vi "Main.vi"(11 "Module Admin":refnum<class "Delacor_lib_QMH_Module Admin.lvclass">) -> ()   [LabVIEW 2020, in "Control Property Tree.lvlib"]
doc: "This template is based off of the Queued Message Handler design pattern and the Queued Message Handler project template that ships with LabVIEW.\n\nThe main difference is that the queue is private to this module and communication between modules is performed via Broadcast and Request events.\n\nRequest events are wrapped in public API methods and are handled in the Event Handling Loop (EHL) of this VI. Any module can register for Broadcast events sent by this module. The EHL generates messages based on user interface actions.\n\nThe Message Handling Loop (MHL) processes messages generated by the EHL, or by other messages. The messages are string values, so new messages can be added easily to the Message Cases case structure in the MHL. Each message cluster can also provide an optional value for Message Data, which is a variant that can be converted to whatever message-specific data is required.\n_____\nBased on Delacor QMH Project Template 5.0.0.82."
uses:
  Control Property Tree.lvlib
  <vilib>/Delacor/Delacor QMH/Libraries/Module Admin_class/Delacor_lib_QMH_Module Admin.lvclass
  Module Data--cluster.ctl
  <vilib>/Delacor/Delacor QMH/Libraries/Message Queue_class/Delacor_lib_QMH_Message Queue.lvclass/Delacor_lib_QMH_Message Queue.ctl
  Stop Argument--cluster.ctl
  <vilib>/Delacor/Delacor QMH/Libraries/Module Admin_class/Delacor_lib_QMH_Module Admin.lvclass/Delacor_lib_QMH_Module Admin.ctl
  Load Available PN Argument--cluster.ctl
  <vilib>/Utility/miscctls.llb/LVPointTypeDef.ctl
  <vilib>/Delacor/Delacor QMH/Libraries/Message Queue_class/Delacor_lib_QMH_Enqueue Message (Single).vi
  <vilib>/Delacor/Delacor QMH/Libraries/Module Admin_class/Delacor_lib_QMH_Get External Launch.vi
  <vilib>/Utility/error.llb/Error Cluster From Error Code.vi
  <vilib>/ErrorRing/Error Ring.xnode
  <vilib>/Delacor/Delacor QMH/Libraries/Message Queue_class/Delacor_lib_QMH_Message Queue.lvclass
panel:
  in  "Add Control":bool
  in  "Remove Control":bool
  in  "List of Controls":string[](tree)
  in  "List of Properties":string(tree)
  in  "Simulate MHL Error":bool
  in  "Simulate EHL Error":bool
  out "error out":errorcluster
  out "Status":string
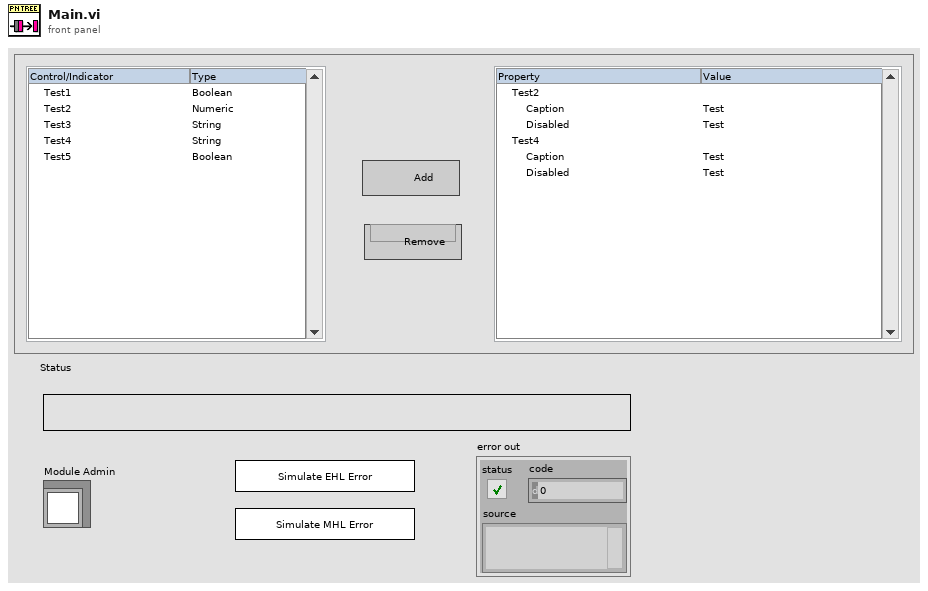
[diagram p1: front panel]
types:
  T1 = typedef "Control Property Tree.lvlib/Request Events--cluster.ctl" = cluster{"Stop Module":refnum<user-event>, "Show Panel":refnum<user-event>, "Hide Panel":refnum<user-event>, "Get Module Execution Status":refnum<user-event>, "Show Diagram":refnum<user-event>, "Load List of Controls":refnum<user-event>, "Load Available PN":refnum<user-event>}
  T2 = typedef "Control Property Tree.lvlib/Module Data--cluster.ctl" = cluster{"Status":string, "UI Ctrls":cluster{"Ctrl Names":string[], "Ctrl Types":string[], "Ctrl Tags":string[]}, "Selected Ctrls":cluster{"Ctrl Names":string[], "Ctrl Types":string[], "Ctrl Tags":string[]}, "Ctrl Properties":map{string, cluster{"Name":string, "Type":string, "Properties":cluster{"Property name":string, "Property value":variant}[]}}, "Ctrl Properties Template":map{string, cluster{"Property name":string, "Property value":variant}[]}}
  T3 = enum32{"invalid lock state", "Not Locked", "Locked (No Password)", "Password-protected"}
  T4 = typedef "Control Property Tree.lvlib/Stop Argument--cluster.ctl" = cluster{"Origin":string, "Exit via Stop Module Req?":bool, "Wait for Module to stop?":bool}
  T5 = typedef "Control Property Tree.lvlib/Load Available PN Argument--cluster.ctl" = cluster{"Boolean":bool}
  T6 = typedef "LVPointTypeDef.ctl" = cluster{"Horizontal":i16, "Vertical":i16}
  T7 = enum32{"Invalid", "Standard", "Closed", "Hidden", "Minimized", "Maximized"}
  T8 = cluster{"Ctrl Names":string[], "Ctrl Types":string[], "Ctrl Tags":string[]}
  T9 = cluster{"Property name":string, "Property value":variant}[]
  T10 = map{string, cluster{"Property name":string, "Property value":variant}[]}
  T11 = cluster{"Left Cell String":string, "Child Text":string[], "Child Tag":string, "Item Indent":i32, "Child Only?":bool, "Glyph Index":i32}[]
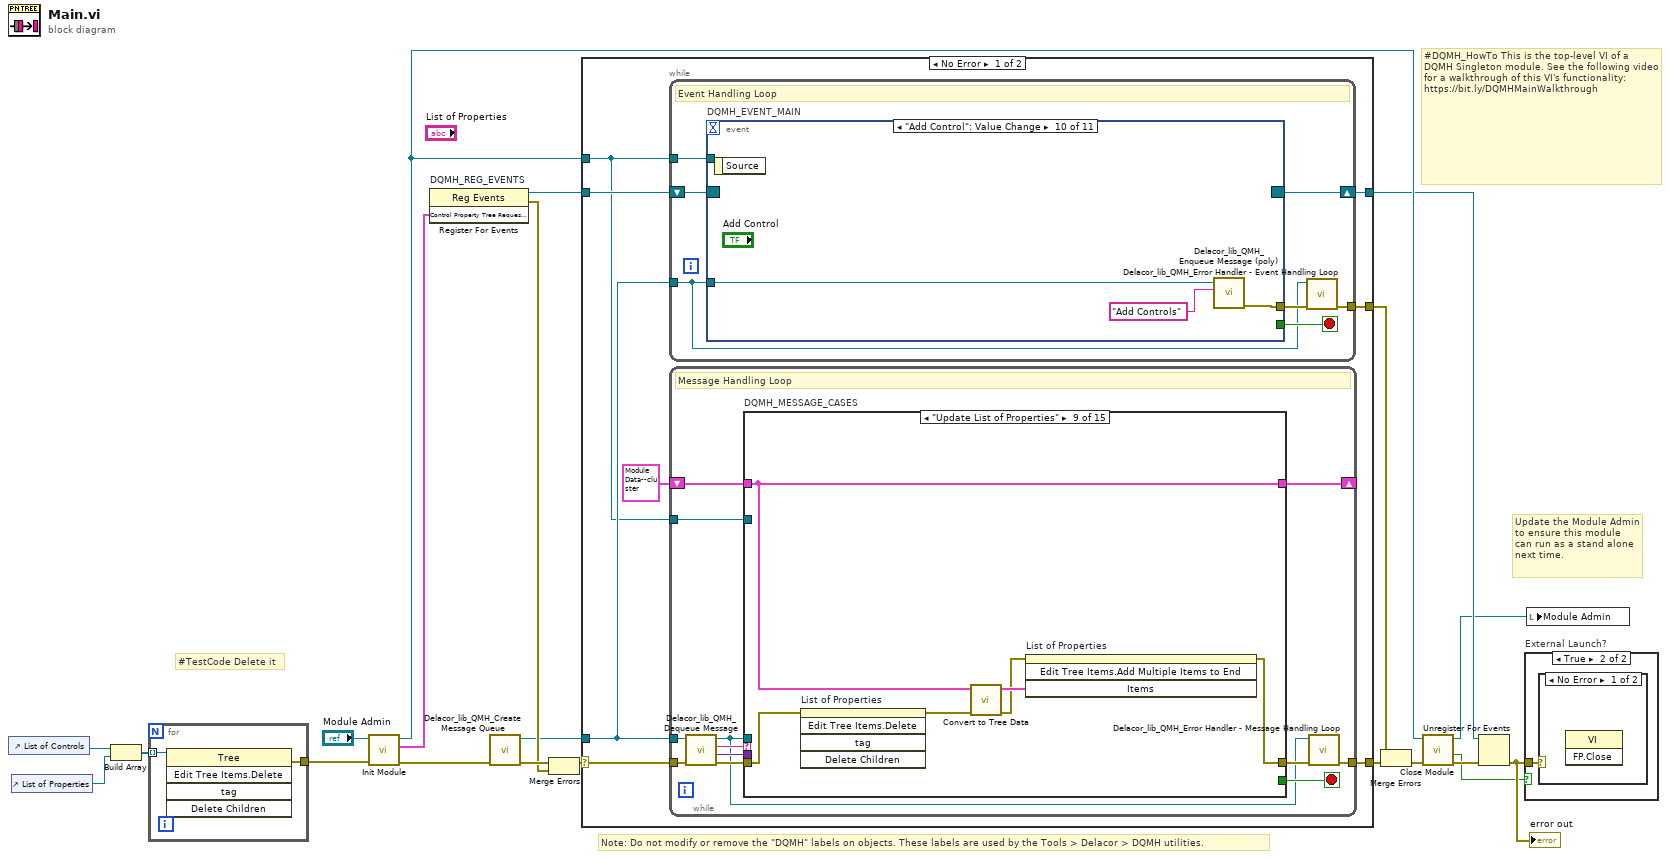
[diagram p0: block diagram]
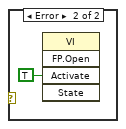
[diagram p3: hidden frame]
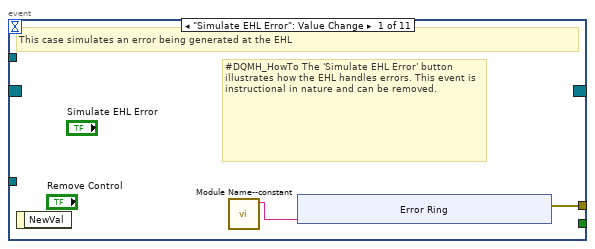
[diagram p4: hidden frame]
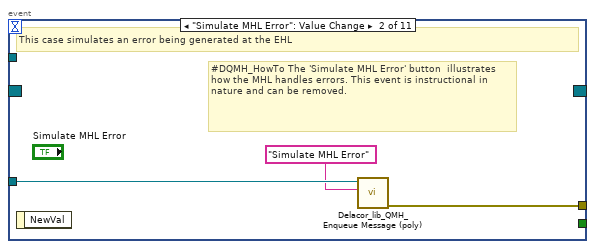
[diagram p5: hidden frame]
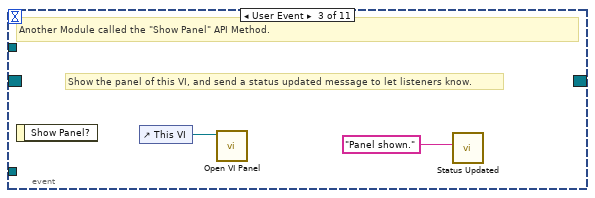
[diagram p6: hidden frame]
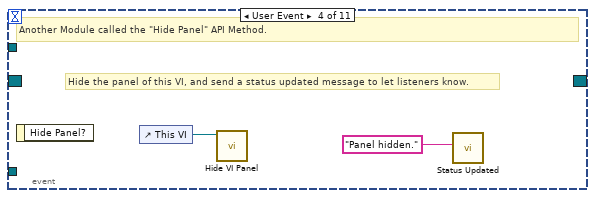
[diagram p7: hidden frame]
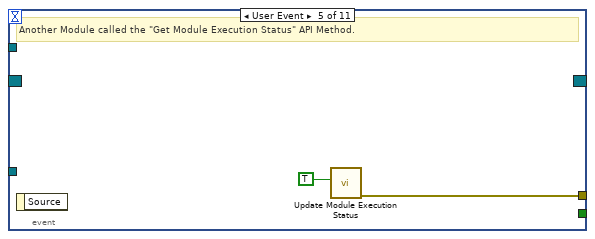
[diagram p8: hidden frame]
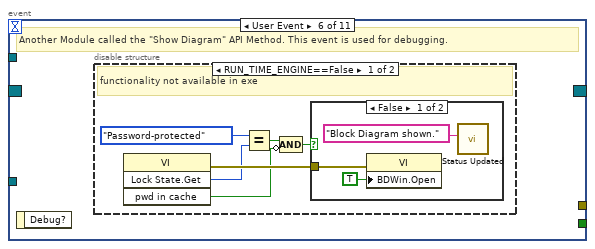
[diagram p9: hidden frame]
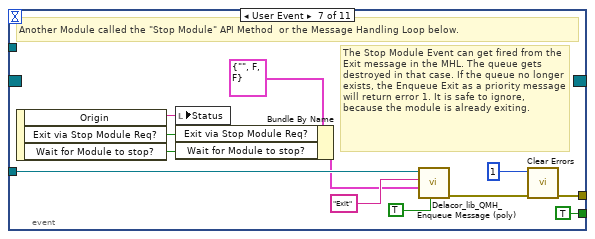
[diagram p12: hidden frame]
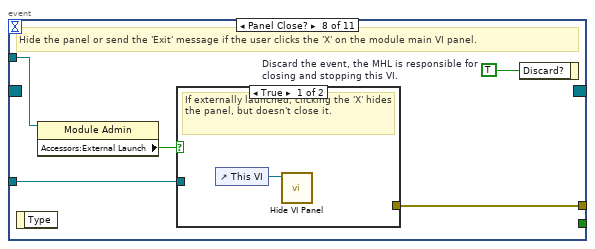
[diagram p13: hidden frame]
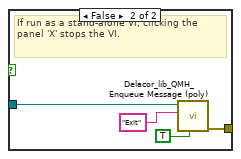
[diagram p14: hidden frame]
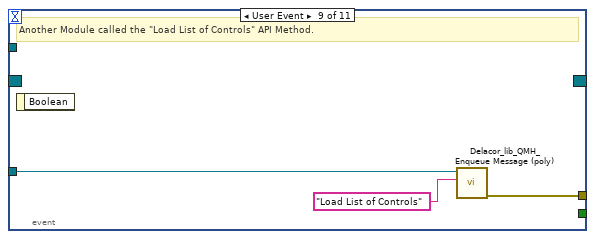
[diagram p15: hidden frame]
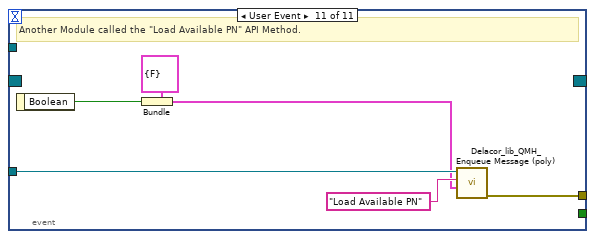
[diagram p16: hidden frame]
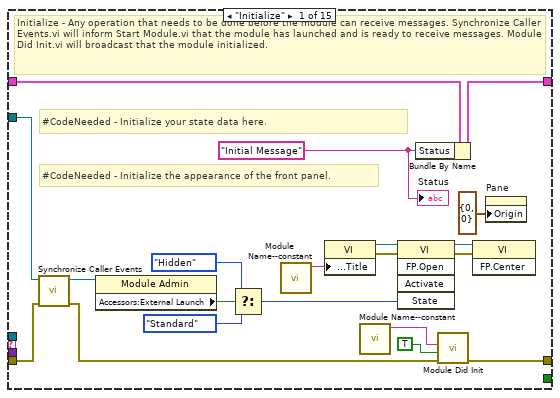
[diagram p17: hidden frame]
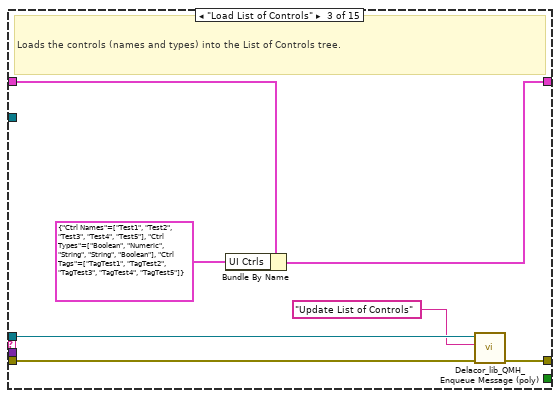
[diagram p19: hidden frame]
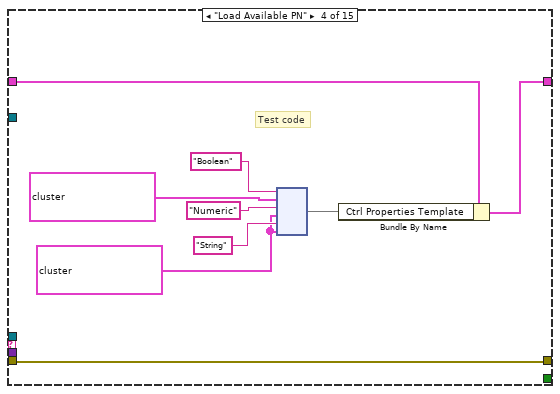
[diagram p20: hidden frame]
diagram:
  # "#TestCode Delete it"
  # "#DQMH_HowTo This is the top-level VI of a DQMH Singleton module. See the following video for a walkthrough of this VI's functionality: https://bit.ly/DQMHMainWalkthrough"
  # "Note: Do not modify or remove the \"DQMH\" labels on objects. These labels are used by the Tools > Delacor > DQMH utilities."
  # "Update the Module Admin to ensure this module can run as a stand alone next time."
  n1 = control-ref of="List of Controls"() -> (w3:refnum<vi>)
  n2 = control-ref of="List of Properties"() -> (w2:refnum<vi>)
  n3 = Build Array(w3, w2) -> (w1:refnum<vi>[])
  n4 = for {
    tunnel: [w23] -> w4
    tunnel: w1 -> [w22] mode=indexing
    n5 = invoke on="Invoke Node" class="Tree" method="Edit Tree Items.Delete"(reference=w22) -> (error out=w23:errorcluster)  [unwired: 4 in, 4 out]
  }
  n6 = call "Init Module.vi"("error in (no error)"=w4, "Singleton Module Admin in"="Module Admin") -> ("error out"=w20:errorcluster, "Control Property Tree Request Events"=w9:T1, "Singleton Module Admin out"=w12:refnum<class "Delacor_lib_QMH_Module Admin.lvclass">)  [unwired: 7 in]
  n7 = register-events "DQMH_REG_EVENTS"(w9) -> (reference out=w10:refnum<event-registration>, error out=w13:errorcluster)  [unwired: 2 in]
  n8 = call <vilib>:"Delacor_lib_QMH_Create Message Queue.vi"("error in (no error)"=w20) -> ("error out"=w15:errorcluster, "Message Queue"=w8:refnum<class "Delacor_lib_QMH_Message Queue.lvclass">)  [unwired: 9 in]
  n9 = Merge Errors(w15, w13) -> (w14:errorcluster)
  n10 = case shown="No Error" w14 {
    selector: w14 -> [w29 w246]
    tunnel: [w31 w245] -> w21
    tunnel: [w28 w251] -> w11
    tunnel: w10 -> [w26 w251]
    tunnel: w8 -> [w25 w244]
    tunnel: [w30 _] -> w18
    tunnel: w12 -> [w24 w247]
    frame No Error {
      n11 = while {
        tunnel: w25 -> [w32]
        shift-right: [w35] -> w28
        shift-left: w26 -> [w36]
        tunnel: [w37] -> w30
        tunnel: w24 -> [w33]
        stop <- w34 stop-if-true
        # "Event Handling Loop"
        n12 = event "DQMH_EVENT_MAIN" shown="[9] \"Add Control\": Value Change" {
          selector: w36 -> [_ _ _ _ _ _ _ _ _ _ _]
          dyn-events: [_ _ _ _ _ _ _ _ _ _ _] -> w35
          timeout: _ -> [_ _ _ _ _ _ _ _ _ _ _]
          tunnel: [_ _ _ _ _ _ TRUE ("Discard?") _ _ _ _] -> w34
          tunnel: w32 -> [_ w49 _ _ _ _ w73 w80 w90 w92 w99]
          tunnel: [w40 w50 _ _ w56 _ w76 w82 w88 w91 w94] -> w38
          tunnel: w33 -> [_ _ _ _ _ _ _ w79 _ _ _]
          event "Simulate EHL Error": Value Change {
            # "#DQMH_HowTo The 'Simulate EHL Error' button  illustrates how the EHL handles errors. This event is instructional in nature and can be removed."
            # "This case simulates an error being generated at the EHL"
            n13 = event-data() -> ()  [unwired: 1 in, 1 out]
            n14 = call "Module Name--constant.vi"() -> ("Module Name"=w39:string)  [unwired: 11 in]
            n15 = xnode "Error Ring"("parameter 0"=w39) -> ("error out"=w40:errorcluster)
          }
          event "Simulate MHL Error": Value Change {
            # "#DQMH_HowTo The 'Simulate MHL Error' button  illustrates how the MHL handles errors. This event is instructional in nature and can be removed."
            # "This case simulates an error being generated at the EHL"
            n16 = event-data() -> ()  [unwired: 1 in, 1 out]
            n17 = call-poly <vilib>:"Delacor_lib_QMH_Enqueue Message (poly).vi"("Message"="Simulate MHL Error", "Message Queue in"=w49) -> ("error out"=w50:errorcluster)  [unwired: 8 in, 1 out]
          }
          event User Event {
            # "Show the panel of this VI, and send a status updated message to let listeners know."
            # "Another Module called the \"Show Panel\" API Method."
            n18 = event-data() -> ()  [unwired: 1 in, 1 out]
            n19 = control-ref of="This VI"() -> (w52:refnum<vi>)
            n20 = call "Open VI Panel.vi"("VI"=w52) -> ()  [unwired: 10 in, 1 out]
            n21 = call "Status Updated.vi"("Status"="Panel shown." ("format string")) -> ()  [unwired: 10 in, 1 out]
          }
          event User Event {
            # "Hide the panel of this VI, and send a status updated message to let listeners know."
            # "Another Module called the \"Hide Panel\" API Method."
            n22 = event-data() -> ()  [unwired: 1 in, 1 out]
            n23 = control-ref of="This VI"() -> (w54:refnum<vi>)
            n24 = call "Hide VI Panel.vi"("VI"=w54) -> ()  [unwired: 10 in, 1 out]
            n25 = call "Status Updated.vi"("Status"="Panel hidden." ("format string")) -> ()  [unwired: 10 in, 1 out]
          }
          event User Event {
            # "Another Module called the \"Get Module Execution Status\" API Method."
            n26 = event-data() -> ()  [unwired: 1 in, 1 out]
            n27 = call "Update Module Execution Status.vi"("Running?"=TRUE) -> ("error out"=w56:errorcluster)  [unwired: 10 in]
          }
          event User Event {
            # "Another Module called the \"Show Diagram\" API Method. This event is used for debugging."
            n28 = event-data() -> ()  [unwired: 1 in, 1 out]
            n29 = disable-structure shown="RUN_TIME_ENGINE==False" {
              frame condition #0 (active) {
                # "functionality not available in exe"
                n30 = invoke class="VI" method="Lock State.Get"() -> (error out=w62:errorcluster, "Get Lock State"=w61:T3, "pwd in cache"=w58:bool)  [unwired: 4 in, 1 out]
                n31 = Equal?(x=T3."Password-protected", y=w61) -> (x = y?=w59:bool)
                n32 = Compound Arithmetic op=AND(w59, invert w58) -> (w57:bool)
                n33 = case shown="False" w57 {
                  tunnel: w62 -> [w65 _]
                  frame False {
                    n34 = property class="VI"(error in=w65, "BDWin.Open"=TRUE ("Block Diagram Window:Open")) -> ()  [unwired: 1 in, 2 out]
                    n35 = call "Status Updated.vi"("Status"="Block Diagram shown." ("format string")) -> ()  [unwired: 10 in, 1 out]
                  }
                  frame True {
                    # "Password-protected VI, and the password is not in the cache. Do not show the diagram."
                  }
                }
              }
              frame condition #1 {
              }
            }
          }
          event User Event {
            # "The Stop Module Event can get fired from the Exit message in the MHL. The queue gets destroyed in that case. If the queue no longer exists, the Enqueue Exit as a priority message will return error 1. It is safe to ignore, because the module is already exiting."
            # "Another Module called the \"Stop Module\" API Method  or the Message Handling Loop below."
            n36 = event-data() -> ("Origin"=w72:string, "Exit via Stop Module Req?"=w68:bool, "Wait for Module to stop?"=w67:bool)  [unwired: 1 in]
            n37 = local write "Status"(w72) -> ()
            n38 = Bundle By Name(cluster=T4 {"Origin"="", "Exit via Stop Module Req?"=FALSE, "Wait for Module to stop?"=FALSE} ("Stop Argument"), "Exit via Stop Module Req?"=w68, "Wait for Module to stop?"=w67) -> (w66:T4)
            n39 = call-poly <vilib>:"Delacor_lib_QMH_Enqueue Message (poly).vi"("Priority Message? (F)"=TRUE, "Message Data"=w66, "Message"="Exit", "Message Queue in"=w73) -> ("error out"=w77:errorcluster)  [unwired: 6 in, 1 out]
            n40 = call <vilib>:"Clear Errors.vi"("error in (no error)"=w77, "specific error code to clear (0: all)"=1) -> ("error out"=w76:errorcluster)  [unwired: 4 in, 1 out]
          }
          event Panel Close? {
            w81 = TRUE  # Discard the event, the MHL is responsible for closing and stopping this VI.
            # "Hide the panel or send the 'Exit' message if the user clicks the 'X' on the module main VI panel."
            n41 = event-data() -> ()  [unwired: 1 in, 1 out]
            n42 = property class="Module Admin"(reference=w79) -> ("Accessors:External Launch"=w78:bool)  [unwired: 1 in, 2 out]
            n43 = case shown="True" w78 {
              tunnel: w80 -> [_ w86]
              tunnel: [_ w87] -> w82
              frame True {
                # "If externally launched, clicking the 'X' hides the panel, but doesn't close it."
                n44 = control-ref of="This VI"() -> (w83:refnum<vi>)
                n45 = call "Hide VI Panel.vi"("VI"=w83) -> ()  [unwired: 10 in, 1 out]
              }
              frame False {
                # "If run as a stand-alone VI, clicking the panel 'X' stops the VI."
                n46 = call-poly <vilib>:"Delacor_lib_QMH_Enqueue Message (poly).vi"("Priority Message? (F)"=TRUE, "Message"="Exit", "Message Queue in"=w86) -> ("error out"=w87:errorcluster)  [unwired: 7 in, 1 out]
              }
            }
            n47 = event-data("Discard?"=w81) -> ()  [unwired: 1 in, 1 out]
          }
          event User Event {
            # "Another Module called the \"Load List of Controls\" API Method."
            n48 = event-data() -> ()  [unwired: 1 in, 1 out]
            n49 = call-poly <vilib>:"Delacor_lib_QMH_Enqueue Message (poly).vi"("Message"="Load List of Controls", "Message Queue in"=w90) -> ("error out"=w88:errorcluster)  [unwired: 8 in, 1 out]
          }
          event "Add Control": Value Change {
            n50 = event-data() -> ()  [unwired: 1 in, 1 out]
            n51 = call-poly <vilib>:"Delacor_lib_QMH_Enqueue Message (poly).vi"("Message"="Add Controls", "Message Queue in"=w92) -> ("error out"=w91:errorcluster)  [unwired: 8 in, 1 out]
          }
          event User Event {
            # "Another Module called the \"Load Available PN\" API Method."
            n52 = event-data() -> ("Boolean"=w95:bool)  [unwired: 1 in]
            n53 = Bundle(cluster=T5 {"Boolean"=FALSE} ("Load Available PN Argument"), "Boolean"=w95) -> (w96:T5)
            n54 = call-poly <vilib>:"Delacor_lib_QMH_Enqueue Message (poly).vi"("Message Data"=w96, "Message"="Load Available PN", "Message Queue in"=w99) -> ("error out"=w94:errorcluster)  [unwired: 7 in, 1 out]
          }
        }
        n55 = call-dynamic "Delacor_lib_QMH_Error Handler - Event Handling Loop.vi"("error in (no error)"=w38, "Message Queue in"=w32) -> ("dup error in"=w37:errorcluster)  [unwired: 8 in, 1 out]
      }
      n56 = while {
        tunnel: w25 -> [w102]
        shift-right: [w106] -> _
        shift-left: T2 {"Status"="", "UI Ctrls"={"Ctrl Names"=[], "Ctrl Types"=[], "Ctrl Tags"=[]}, "Selected Ctrls"={"Ctrl Names"=[], "Ctrl Types"=[], "Ctrl Tags"=[]}, "Ctrl Properties"={}, "Ctrl Properties Template"={}} ("Data Cluster") -> [w107]
        tunnel: w29 -> [w110]
        tunnel: [w108] -> w31
        tunnel: w24 -> [w100]
        stop <- w105 stop-if-true
        # "Message Handling Loop"
        n57 = call-dynamic "Delacor_lib_QMH_Dequeue Message.vi"("error in (no error)"=w110, "Message Queue in"=w102) -> ("error out"=w109:errorcluster, "Message Data"=w103:variant, "Message"=w104:string, "Message Queue out"=w101:refnum<class "Delacor_lib_QMH_Message Queue.lvclass">)  [unwired: 6 in]
        n58 = case "DQMH_MESSAGE_CASES" shown="\"Update List of Properties\"" w104 {
          selector: w104 -> [_ _ _ _ _ _ _ _ _ _ _ _ _ _ w231]
          tunnel: w101 -> [_ _ w135 _ _ w155 _ w171 _ _ _ _ w201 w223 _]
          tunnel: w109 -> [w129 w133 w137 w141 w151 w160 w164 w170 w176 w183 w185 w190 w208 w229 w233]
          tunnel: [w127 w133 w136 w141 w154 w156 w163 w169 w180 w182 w185 w189 w204 w226 w234] -> w111
          tunnel: w107 -> [w118 w132 w140 w143 w153 w162 w167 w174 w179 w181 w184 w187 w203 w222 w232]
          tunnel: [w117 w132 w138 w142 w153 w162 w166 w173 w179 w181 w184 w187 w203 w222 w232] -> w106
          tunnel: [_ _ _ _ _ _ _ _ _ _ _ _ _ w221 _] -> w105
          tunnel: w103 -> [_ _ _ _ _ _ _ _ _ _ _ _ w202 w220 _]
          tunnel: w100 -> [w119 _ _ _ _ _ _ _ _ _ _ _ w200 w215 _]
          frame "Initialize" {
            w112 = "Initial Message" ("Initial Message")
            # "#CodeNeeded - Initialize the appearance of the front panel."
            # "#CodeNeeded - Initialize your state data here."
            # "Initialize - Any operation that needs to be done before the module can receive messages. Synchronize Caller Events.vi will inform Start Module.vi that the module has launched and is ready to receive messages. Module Did Init.vi will broadcast that the module initialized."
            n59 = call "Synchronize Caller Events.vi"("error in (no error)"=w129, "Singleton Module Admin in"=w119) -> ("error out"=w128:errorcluster, "Singleton Module Admin out"=w114:refnum<class "Delacor_lib_QMH_Module Admin.lvclass">)  [unwired: 8 in]
            n60 = property class="Module Admin"(reference=w114) -> ("Accessors:External Launch"=w123:bool)  [unwired: 1 in, 2 out]
            n61 = Select(t=T7."Hidden" ("State"), s=w123, f=T7."Standard" ("State")) -> (s? t:f=w120:T7)
            n62 = call "Module Name--constant.vi"() -> ("Module Name"=w126:string)  [unwired: 11 in]
            n63 = property class="VI"("Front Panel.Title"=w126) -> (reference out=w125:refnum<vi>, error out=w131:errorcluster)  [unwired: 2 in]
            n64 = call "Module Name--constant.vi"() -> ("Module Name"=w115:string)  [unwired: 11 in]
            n65 = invoke class="VI" method="FP.Open"(reference=w125, error in=w131, "State"=w120) -> (reference out=w124:refnum<vi>, error out=w130:errorcluster)  [unwired: 2 in, 3 out]
            n66 = Bundle By Name(cluster=w118, "Status"=w112) -> (w117:T2)
            n67 = call "Module Did Init.vi"("error in (no error)"=w128, "Initialized?"=TRUE, "Origin"=w115) -> ("error out"=w127:errorcluster)  [unwired: 8 in]
            n68 = invoke class="VI" method="FP.Center"(reference=w124, error in=w130) -> ()  [unwired: 1 in, 3 out]
            n69 = property on="Pane" class="Pane"("Origin"=T6 {"Horizontal"=0, "Vertical"=0}) -> ()  [unwired: 2 in, 2 out]
            "Status" <- w112
          }
          frame "--- Module Specific ---" {
            # "Separator -- The following cases handle messages specific to this Module."
          }
          frame "Load List of Controls" {
            # "Loads the controls (names and types) into the List of Controls tree."
            n70 = Bundle By Name(cluster=w140, "UI Ctrls"=T8 {"Ctrl Names"=["Test1", "Test2", "Test3", "Test4", "Test5"], "Ctrl Types"=["Boolean", "Numeric", "String", "String", "Boolean"], "Ctrl Tags"=["TagTest1", "TagTest2", "TagTest3", "TagTest4", "TagTest5"]}) -> (w138:T2)
            n71 = call-poly <vilib>:"Delacor_lib_QMH_Enqueue Message (poly).vi"("error in (no error)"=w137, "Message"="Update List of Controls", "Message Queue in"=w135) -> ("error out"=w136:errorcluster)  [unwired: 7 in, 1 out]
          }
          frame "Load Available PN" {
            w145 = T9 [{"Property name"="Caption", "Property value"=variant}, {"Property name"="Disabled", "Property value"=variant}] ("Properties")
            # "Test code"
            n72 = node("Boolean" ("key"), T9 [{"Property name"="Caption", "Property value"=variant}, {"Property name"="Disabled", "Property value"=variant}, {"Property name"="Blinking", "Property value"=variant}] ("Properties"), "Numeric" ("key"), w145, "String" ("key"), w145) -> (w144:T10)
            n73 = Bundle By Name(cluster=w143, "Ctrl Properties Template"=w144) -> (w142:T2)
          }
          frame "Update List of Controls" {
            n74 = call "Update List of Controls Tree.vi"("error in (no error)"=w151, "Data Cluster"=w153) -> ("error out"=w150:errorcluster, "Items"=w152:T11)  [unwired: 8 in]
            n75 = invoke on="List of Controls" class="Tree (strict)" method="Edit Tree Items.Add Multiple Items to End"(error in=w150, "Items"=w152) -> (error out=w154:errorcluster)  [unwired: 2 in, 3 out]
          }
          frame "Add Controls" {
            n76 = call-poly <vilib>:"Delacor_lib_QMH_Enqueue Message (poly).vi"("error in (no error)"=w160, "Message"="Read Selected Controls", "Message Queue in"=w155) -> ("error out"=w158:errorcluster, "Message Queue out"=w157:refnum<class "Delacor_lib_QMH_Message Queue.lvclass">)  [unwired: 7 in]
            n77 = call-poly <vilib>:"Delacor_lib_QMH_Enqueue Message (poly).vi"("error in (no error)"=w158, "Message"="Add to Ctrl Properties", "Message Queue in"=w157) -> ("error out"=w156:errorcluster)  [unwired: 7 in, 1 out]
          }
          frame "Read Selected Controls" {
            n78 = call "Get Selected Controls.vi"("error in (no error)"=w164, "List of Controls"="List of Controls", "Data in"=w167) -> ("error out"=w163:errorcluster, "Selected Ctrls"=w165:T8)  [unwired: 7 in]
            n79 = Bundle By Name(cluster=w167, "Selected Ctrls"=w165) -> (w166:T2)
          }
          frame "Add to Ctrl Properties" {
            n80 = call "Add Selected Ctrl Properties.vi"("Data Cluster In"=w174) -> ("Data Cluster out"=w173:T2)
            n81 = call-poly <vilib>:"Delacor_lib_QMH_Enqueue Message (poly).vi"("error in (no error)"=w170, "Message"="Update List of Properties", "Message Queue in"=w171) -> ("error out"=w169:errorcluster)  [unwired: 7 in, 1 out]
          }
          frame "Update List of Properties" {
            n82 = invoke on="List of Properties" class="Tree (strict)" method="Edit Tree Items.Delete"(error in=w176) -> (error out=w175:errorcluster)  [unwired: 4 in, 4 out]
            n83 = call "Convert to Tree Data.vi"("error in (no error)"=w175, "Data Cluster"=w179) -> ("error out"=w177:errorcluster, "Items out"=w178:T11)  [unwired: 8 in]
            n84 = invoke on="List of Properties" class="Tree (strict)" method="Edit Tree Items.Add Multiple Items to End"(error in=w177, "Items"=w178) -> (error out=w180:errorcluster)  [unwired: 2 in, 3 out]
          }
          frame "---Copy This Frame---" {
            # "Duplicate this frame when creating new messages.  Change this comment in the duplicated frame to describe this message."
            n85 = Merge Errors(w183) -> (w182:errorcluster)
          }
          frame "--- Exit and Error Handling---" {
            # "Separator - The following cases handle errors and exit messages."
          }
          frame "Simulate MHL Error" {
            # "#DQMH_HowTo The 'Simulate MHL Error' button  illustrates how the MHL handles errors. This event is instructional in nature and can be removed."
            # "Simulate an error occurring at the MHL"
            n86 = call "Module Name--constant.vi"() -> ("Module Name"=w186:string)  [unwired: 11 in]
            n87 = xnode "Error Ring"("parameter 0"=w186) -> ("error out"=w188:errorcluster)
            n88 = Merge Errors(w190, w188) -> (w189:errorcluster)
          }
          frame "Error" {
            # "#CodeRecommended - If you ever change the name of this \"Error\" message, you'll need to update the name in the Check Loop Error.vi as well."
            # "#CodeRecommended - If the module is running in standalone mode (External Launch = FALSE), this code will pop up an error dialog and call the 'Exit' message if an error occurs. Add more fine-grained error handling here."
            # "Error - Check the error message data and respond accordingly. This message is sent by the \"Error Handler\" VIs at the end of each loop in this application."
            n89 = property class="Module Admin"(reference=w200) -> ("Accessors:External Launch"=w199:bool)  [unwired: 1 in, 2 out]
            n90 = Variant To Data(error in=w208, type=errorcluster {"status"=FALSE, "code"=0, "source"=""} ("error constant"), Variant=w202) -> (data=w209:errorcluster, error out=w206:errorcluster)
            n91 = call "Module Name--constant.vi"() -> ("Module Name"=w198:string)  [unwired: 11 in]
            n92 = call "Error Reported.vi"("Additional Information"=w198, "Error"=w209) -> ()  [unwired: 9 in, 1 out]
            n93 = case shown="False" w199 {
              tunnel: [w214 _] -> w205
              tunnel: w201 -> [w212 _]
              tunnel: w209 -> [w213 _]
              frame False {
                # "If the module is running standalone, then pop up an error dialog and call the \"Exit\" message."
                n94 = call <vilib>:"Simple Error Handler.vi"("error in (no error)"=w213) -> ()  [unwired: 4 in, 5 out]
                n95 = call-poly <vilib>:"Delacor_lib_QMH_Enqueue Message (poly).vi"("Priority Message? (F)"=TRUE, "Message"="Exit", "Message Queue in"=w212) -> ("error out"=w214:errorcluster)  [unwired: 7 in, 1 out]
              }
              frame True {
                # "If the module was launched externally, calling the Error Reported broadcast VI is the only action performed by the \"Error\" message. The module's caller can then process the error appropriately."
              }
            }
            n96 = Merge Errors(w206, w205) -> (w204:errorcluster)
            n97 = local write "error out"(w204) -> ()
          }
          frame "Exit" {
            w219 = 91  # 91: not all Exit messages will have an argument
            w221 = TRUE  # Stop the VI
            # "Release the message queue reference"
            # "#CodeNeeded - Add any required cleanup code here"
            # "Exit - Exit the application."
            n98 = Variant To Data(error in=w229, type=T4 {"Origin"="", "Exit via Stop Module Req?"=FALSE, "Wait for Module to stop?"=FALSE} ("Stop Argument"), Variant=w220) -> (data=w217:T4, error out=w225:errorcluster)
            n99 = call <vilib>:"Clear Errors.vi"("error in (no error)"=w225, "specific error code to clear (0: all)"=w219) -> ("error out"=w228:errorcluster)  [unwired: 4 in, 1 out]
            n100 = control-ref of="This VI"() -> (w216:refnum<vi>)
            n101 = call-dynamic "Delacor_lib_QMH_Release Message Queue.vi"("error in (no error)"=w228, "Message Queue"=w223) -> ("error out"=w227:errorcluster)  [unwired: 9 in]
            n102 = call "Handle Exit.vi"("Stop Argument"=w217, "Admin in"=w215, "VI reference"=w216) -> ("error out"=w224:errorcluster)  [unwired: 7 in, 1 out]
            n103 = Merge Errors(w227, w224) -> (w226:errorcluster)
          }
          frame Default {
            # "'Default' case only runs if there is a message that isn't defined in any of the other cases.  Output a programming error."
            n104 = call "Module Name--constant.vi"() -> ("Module Name"=w230:string)  [unwired: 11 in]
            n105 = xnode "Error Ring"("parameter 0"=w231, "parameter 1"=w230) -> ("error out"=w235:errorcluster)
            n106 = Merge Errors(w233, w235) -> (w234:errorcluster)
          }
        }
        n107 = call-dynamic "Delacor_lib_QMH_Error Handler - Message Handling Loop.vi"("error in (no error)"=w111, "Message Queue in"=w101) -> ("dup error in"=w108:errorcluster)  [unwired: 8 in, 1 out]
      }
    }
    frame Error {
      # "Synchronize Caller Events.vi will inform Start Module.vi that the module has launched and will let the code calling Start Module.vi register for broadcasts and would permit the caller receive the broadcast that an error occurred at launch time."
      n108 = call-dynamic "Delacor_lib_QMH_Release Message Queue.vi"("error in (no error)"=w246, "Message Queue"=w244) -> ("error out"=w245:errorcluster)  [unwired: 9 in]
      n109 = call "Synchronize Caller Events.vi"("Singleton Module Admin in"=w247) -> ("error out"=w252:errorcluster)  [unwired: 9 in, 1 out]
      n110 = call "Module Name--constant.vi"() -> ("Module Name"=w250:string)  [unwired: 11 in]
      n111 = Format Into String(format string="An error occurred during initialization. %s is no longer running.", w250) -> (resulting string=w248:string)  [unwired: 2 in, 1 out]
      n112 = Merge Errors(w245, w252) -> (w253:errorcluster)
      n113 = call "Error Reported.vi"("Additional Information"=w248, "Error"=w253) -> ()  [unwired: 9 in, 1 out]
    }
  }
  n114 = Merge Errors(w18, w21) -> (w17:errorcluster)
  n115 = call "Close Module.vi"("error in (no error)"=w17, "Module Admin in"=w12) -> ("error out"=w19:errorcluster, "External Launch"=w5:bool, "Module Admin out"=w6:refnum<class "Delacor_lib_QMH_Module Admin.lvclass">)  [unwired: 7 in]
  n116 = Unregister For Events(event registration refnum=w11, error in=w19) -> (error out=w16:errorcluster)
  "error out" <- w16
  n117 = case "External Launch?" shown="True" w5 {
    tunnel: w16 -> [_ w254]
    frame False {
    }
    frame True {
      n118 = case shown="No Error" w254 {
        frame No Error {
          n119 = invoke class="VI" method="FP.Close"() -> ()  [unwired: 3 in, 3 out]
        }
        frame Error {
          n120 = invoke class="VI" method="FP.Open"("Activate"=TRUE ("Activate?")) -> ()  [unwired: 4 in, 5 out]
        }
      }
    }
  }
  n121 = local write "Module Admin"(w6) -> ()
